vi "KelvinToReomur.vi"(11 "Кельвин":dbl) -> (3 "Реомюр":dbl)   [LabVIEW 2017]
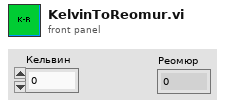
[diagram p1: front panel]
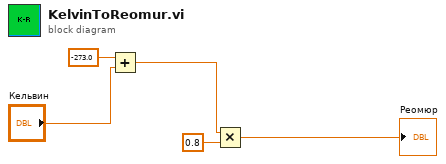
[diagram p0: block diagram]
diagram:
  n1 = Add(x=-273.0, y="Кельвин") -> (x+y=w2:dbl)
  n2 = Multiply(x=w2, y=0.8) -> (x*y=→"Реомюр":dbl)
